vi "TX_Controller.vi"(0 "queue out":refnum<queue>, 1 "DisplayCamera":refnum<user-event>, 2 "StartCamera":refnum<user-event>, 3 "DisCam":refnum<user-event>, 4 "PathLoaded":refnum<user-event>, 5 "TakePhoto":refnum<user-event>, 6 "EnableTCP":refnum<user-event>, 7 "error out":errorcluster, 9 "CloseAll":refnum<user-event>, 11 "CloseAll 2":refnum<user-event>, 13 "CloseAll 3":refnum<user-event>, 15 "CloseAll 4":refnum<user-event>) -> (27 "error out 2":errorcluster)   [LabVIEW 2023]
uses:
  TX_Control 3.ctl
  <vilib>/vision/Image Controls.llb/IMAQ Image.ctl
  <vilib>/userDefined/High Color/IMAQdx.ctl
  <vilib>/vision/driver/NI_Vision_Acquisition_Software.lvlib
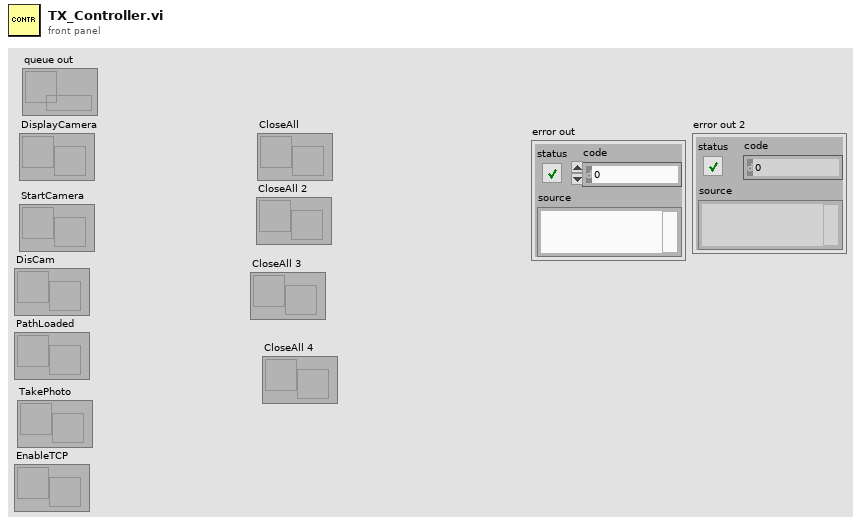
[diagram p1: front panel]
types:
  T1 = typedef "IMAQ Image.ctl" = refnum<image>
  T2 = typedef "IMAQdx.ctl" = refnum<k21>
  T3 = cluster{"skala szaroœci 2":u8, "CamView":T1, "Data":variant, "CamSel":T2, "close":bool}
  T4 = typedef "TX_Control 3.ctl" = enum16{"Default", "PathLoaded", "StartCamera", "TakePhoto", "EnableTCP", "Cam2Display", "CloseAll"}
  T5 = cluster{"Enum":T4, "Data":variant, "Data2":variant}
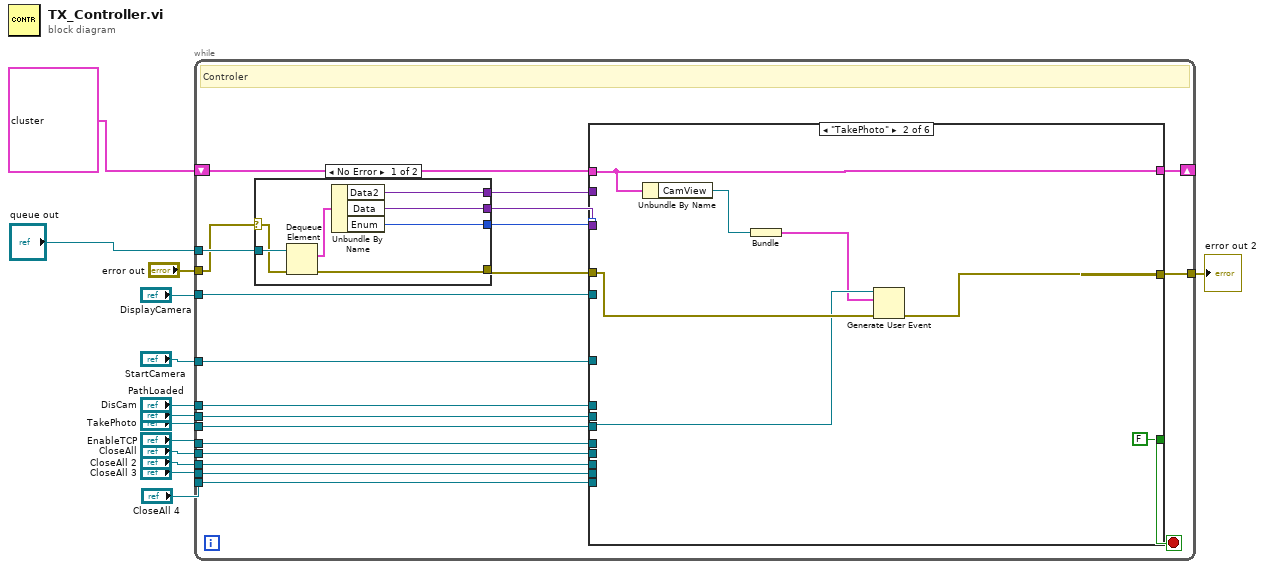
[diagram p0: block diagram]
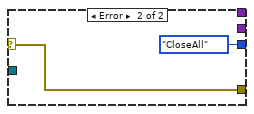
[diagram p2: hidden frame]
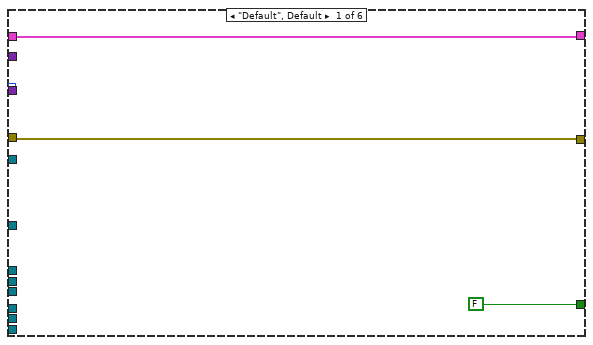
[diagram p3: hidden frame]
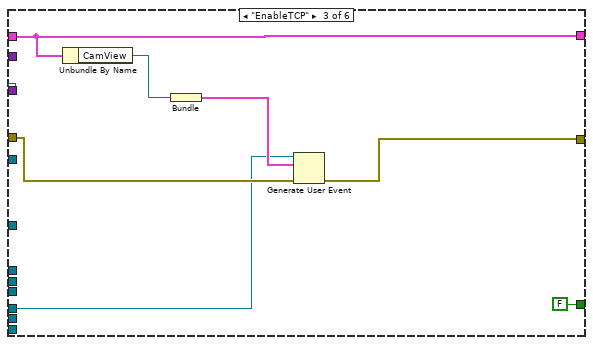
[diagram p4: hidden frame]
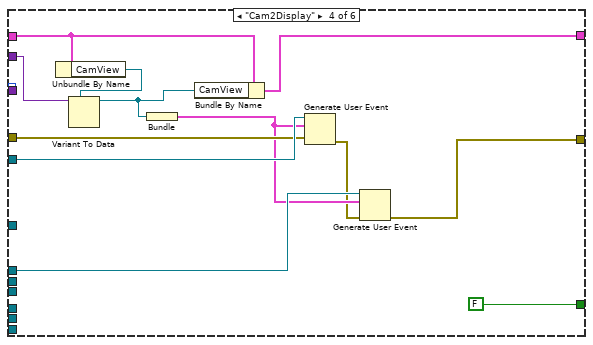
[diagram p5: hidden frame]
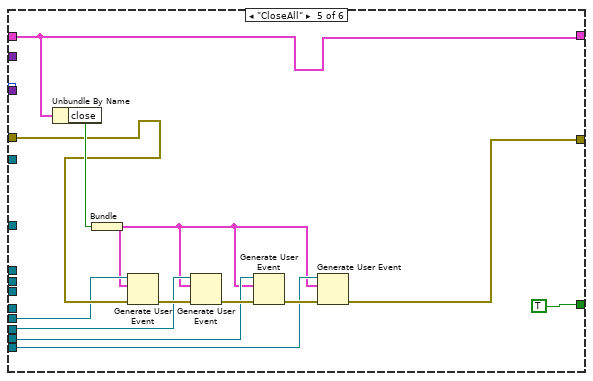
[diagram p6: hidden frame]
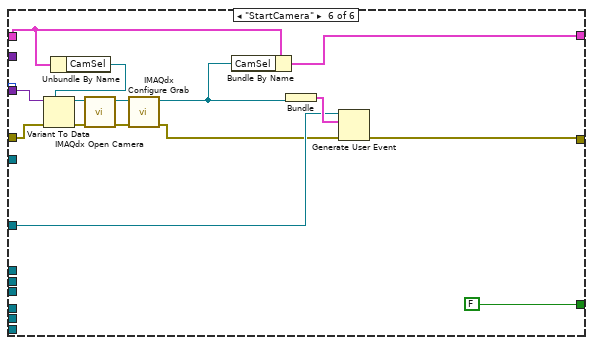
[diagram p7: hidden frame]
diagram:
  n1 = while {
    tunnel: "queue out" -> [w28]
    tunnel: "error out" -> [w19]
    tunnel: "DisplayCamera" -> [w33]
    shift-right: [w31] -> _
    shift-left: T3 {"skala szaroœci 2"=0, "CamView"=refnum, "Data"=variant(refnum<image> refnum), "CamSel"="", "close"=TRUE} ("EditImage") -> [w32]
    tunnel: [w29] -> w1
    tunnel: "PathLoaded" -> [w27]
    tunnel: "StartCamera" -> [w26]
    tunnel: "DisCam" -> [w22]
    tunnel: "TakePhoto" -> [w21]
    tunnel: "EnableTCP" -> [w20]
    tunnel: "CloseAll" -> [w18]
    tunnel: "CloseAll 2" -> [w17]
    tunnel: "CloseAll 3" -> [w16]
    tunnel: "CloseAll 4" -> [w15]
    stop <- w23 stop-if-true
    # "Controler"
    n2 = case shown="No Error" w19 {
      selector: w19 -> [w35 w43]
      tunnel: [w41 TX_Control_3."CloseAll" ("Enum")] -> w34
      tunnel: [w39 w43] -> w30
      tunnel: w28 -> [w38 _]
      tunnel: [w37 _] -> w25
      tunnel: [w36 _] -> w24
      frame No Error {
        n3 = Dequeue Element(queue=w38, error in (no error)=w35) -> (element=w40:T5, error out=w39:errorcluster)  [unwired: 1 in, 2 out]
        n4 = Unbundle By Name(w40) -> ("Data2"=w36:variant, "Data"=w37:variant, "Enum"=w41:T4)
      }
      frame Error {
      }
    }
    n5 = case shown="\"TakePhoto\"" w34 {
      tunnel: w33 -> [_ _ _ w72 _ _]
      tunnel: w32 -> [w46 w49 w57 w69 w82 w99]
      tunnel: [w46 w49 w57 w70 w82 w98] -> w31
      tunnel: w30 -> [w45 w53 w60 w71 w83 w89]
      tunnel: [w45 w51 w59 w61 w78 w100] -> w29
      tunnel: w27 -> [_ _ _ _ _ _]
      tunnel: w26 -> [_ _ _ _ _ w90]
      tunnel: w25 -> [_ _ _ _ _ w95]
      tunnel: w24 -> [_ _ _ w67 _ _]
      tunnel: [FALSE FALSE FALSE FALSE TRUE FALSE] -> w23
      tunnel: w22 -> [_ _ _ w65 _ _]
      tunnel: w21 -> [_ w52 _ _ _ _]
      tunnel: w20 -> [_ _ w54 _ _ _]
      tunnel: w18 -> [_ _ _ _ w77 _]
      tunnel: w17 -> [_ _ _ _ w76 _]
      tunnel: w16 -> [_ _ _ _ w75 _]
      tunnel: w15 -> [_ _ _ _ w74 _]
      frame "Default", Default {
      }
      frame "TakePhoto" {
        n6 = Unbundle By Name(w49) -> ("CamView"=w48:T1)
        n7 = Bundle("CamView"=w48) -> (w47:cluster{"CamView":T1})  [unwired: 1 in]
        n8 = Generate User Event(user event=w52, event data cluster=w47, error in=w53) -> (error out=w51:errorcluster)  [unwired: 1 in, 1 out]
      }
      frame "EnableTCP" {
        n9 = Unbundle By Name(w57) -> ("CamView"=w56:T1)
        n10 = Bundle("CamView"=w56) -> (w55:cluster{"CamView":T1})  [unwired: 1 in]
        n11 = Generate User Event(user event=w54, event data cluster=w55, error in=w60) -> (error out=w59:errorcluster)  [unwired: 1 in, 1 out]
      }
      frame "Cam2Display" {
        n12 = Unbundle By Name(w69) -> ("CamView"=w68:T1)
        n13 = Variant To Data(type=w68, Variant=w67) -> (data=w64:T1)  [unwired: 1 in, 1 out]
        n14 = Bundle("CamView"=w64) -> (w63:cluster{"CamView":T1})  [unwired: 1 in]
        n15 = Bundle By Name(cluster=w69, "CamView"=w64) -> (w70:T3)
        n16 = Generate User Event(user event=w72, event data cluster=w63, error in=w71) -> (error out=w62:errorcluster)  [unwired: 1 in, 1 out]
        n17 = Generate User Event(user event=w65, event data cluster=w63, error in=w62) -> (error out=w61:errorcluster)  [unwired: 1 in, 1 out]
      }
      frame "CloseAll" {
        n18 = Unbundle By Name(w82) -> ("close"=w84:bool)
        n19 = Bundle("close"=w84) -> (w73:cluster{"close":bool})  [unwired: 1 in]
        n20 = Generate User Event(user event=w77, event data cluster=w73, error in=w83) -> (error out=w81:errorcluster)  [unwired: 1 in, 1 out]
        n21 = Generate User Event(user event=w76, event data cluster=w73, error in=w81) -> (error out=w80:errorcluster)  [unwired: 1 in, 1 out]
        n22 = Generate User Event(user event=w75, event data cluster=w73, error in=w80) -> (error out=w79:errorcluster)  [unwired: 1 in, 1 out]
        n23 = Generate User Event(user event=w74, event data cluster=w73, error in=w79) -> (error out=w78:errorcluster)  [unwired: 1 in, 1 out]
      }
      frame "StartCamera" {
        n24 = Unbundle By Name(w99) -> ("CamSel"=w92:T2)
        n25 = Variant To Data(error in=w89, type=w92, Variant=w95) -> (data=w94:T2, error out=w88:errorcluster)
        n26 = call <vilib>:"IMAQdx Open Camera.vi"("error in"=w88, "Session In"=w94) -> ("error out"=w87:errorcluster, "Session Out"=w93:T2)  [unwired: 8 in]
        n27 = call <vilib>:"IMAQdx Configure Grab.vi"("error in"=w87, "Session In"=w93) -> ("error out"=w86:errorcluster, "Session Out"=w91:T2)  [unwired: 8 in]
        n28 = Bundle By Name(cluster=w99, "CamSel"=w91) -> (w98:T3)
        n29 = Bundle("Session Out"=w91) -> (w97:cluster{"Session Out":T2})  [unwired: 1 in]
        n30 = Generate User Event(user event=w90, event data cluster=w97, error in=w86) -> (error out=w100:errorcluster)  [unwired: 1 in, 1 out]
      }
    }
  }
  "error out 2" <- w1
